vi "GetSchedule.vi"(11 "Append to URL":string="CMP") -> (3 "value":T1)   [LabVIEW 2014, in "FIRST Events API.lvlib"]
uses:
  FIRST Events API.lvlib
  FRC Schedule.ctl
  FRC API Selector.ctl
panel:
  out "error out":errorcluster
  out "body":string
  out "headers":string
  out "Generated URL":string
  # "returns the match schedule for the desired tournament level of a particular event in a particular season"
  # "Must contain eventCode"
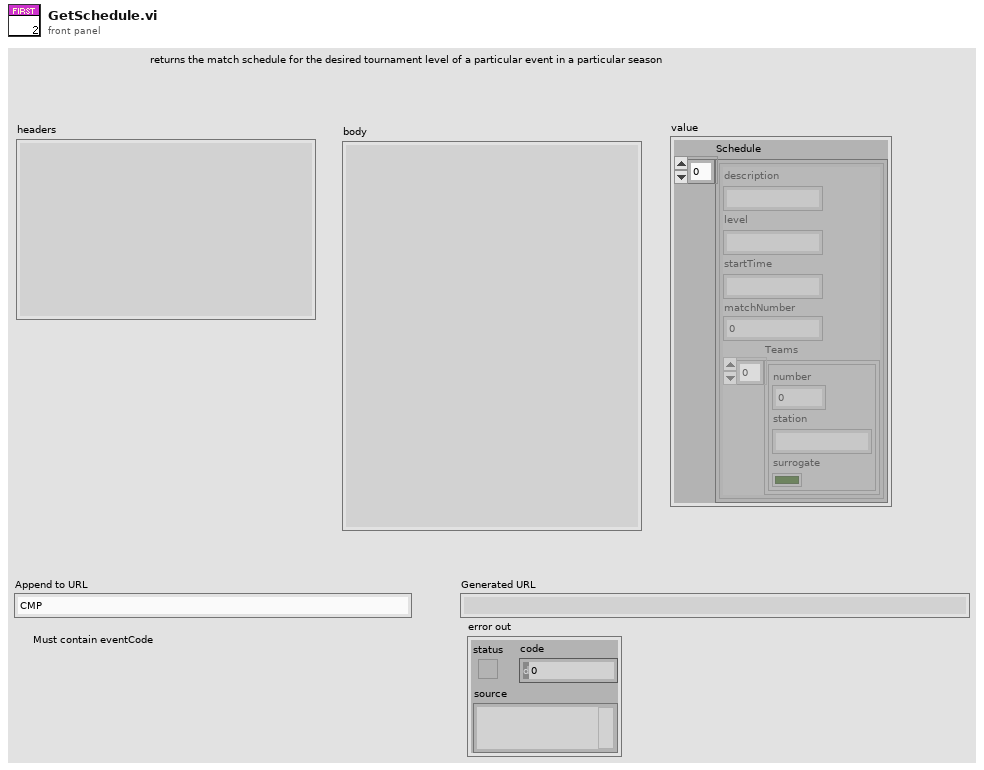
[diagram p1: front panel]
types:
  T1 = typedef "FIRST Events API.lvlib/FRC Schedule.ctl" = cluster{"Schedule":cluster{"description":string, "level":string, "startTime":string, "matchNumber":dbl, "Teams":cluster{"number":dbl, "station":string, "surrogate":bool}[]}[]}
  T2 = typedef "FIRST Events API.lvlib/FRC API Selector.ctl" = enum16{"GetEventAllianceSelection", "Ancillary", "GetTeamListings", "GetSchedule", "GetEventListings"}
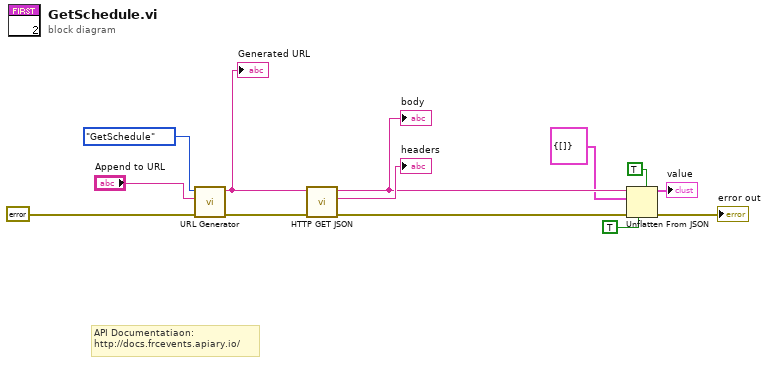
[diagram p0: block diagram]
diagram:
  # "API Documentatiaon:\nhttp://docs.frcevents.apiary.io/"
  n1 = call "URL Generator.vi"("error in (no error)"=errorcluster {"status"=FALSE, "code"=0, "source"=""}, "Append URL"="Append to URL", "API Command"=FRC_API_Selector."GetSchedule") -> ("error out"=w8:errorcluster, "Generated URL"=w11:string)  [unwired: 7 in]
  "Generated URL" <- w11
  n2 = call "HTTP GET JSON.vi"("error in (no error)"=w8, "Generated URL"=w11) -> ("error out"=w6:errorcluster, "headers"=→"headers":string, "body"=w7:string)  [unwired: 7 in]
  "body" <- w7
  n3 = Unflatten From JSON(enable LabVIEW extensions? (T)=TRUE, JSON string=w7, type and defaults=T1 {"Schedule"=[]} ("schedule"), default null elements? (F)=TRUE, error in (no error)=w6) -> (value=→"value":T1, error out=→"error out":errorcluster)  [unwired: 2 in]
